vi "fWform to CSV File.vi"(5 "error in (no error)":errorcluster, 6 "Inlude Time Vector":bool, 7 "wForms":waveform(dbl)[](array[waveform]), 9 "CSV Path IN":path) -> (13 "CSV Path OUT":path, 19 "error out":errorcluster)   [LabVIEW 2020, in "TEXT.lvclass"]
uses:
  TEXT.lvclass
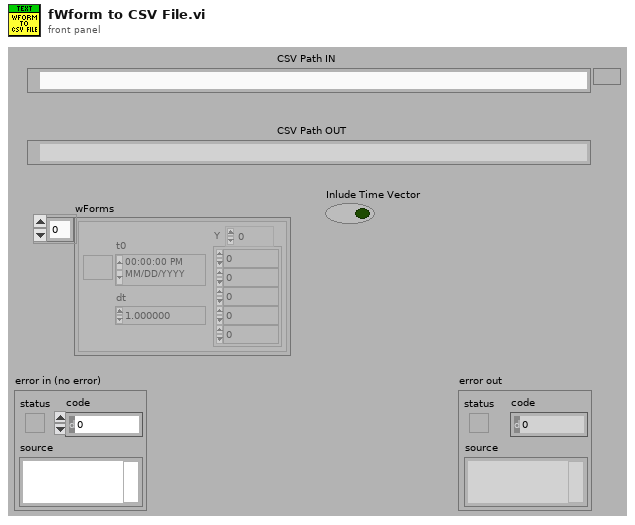
[diagram p1: front panel]
types:
  T1 = enum16{"open", "replace", "create", "open or create", "replace or create", "replace or create with confirmation"}
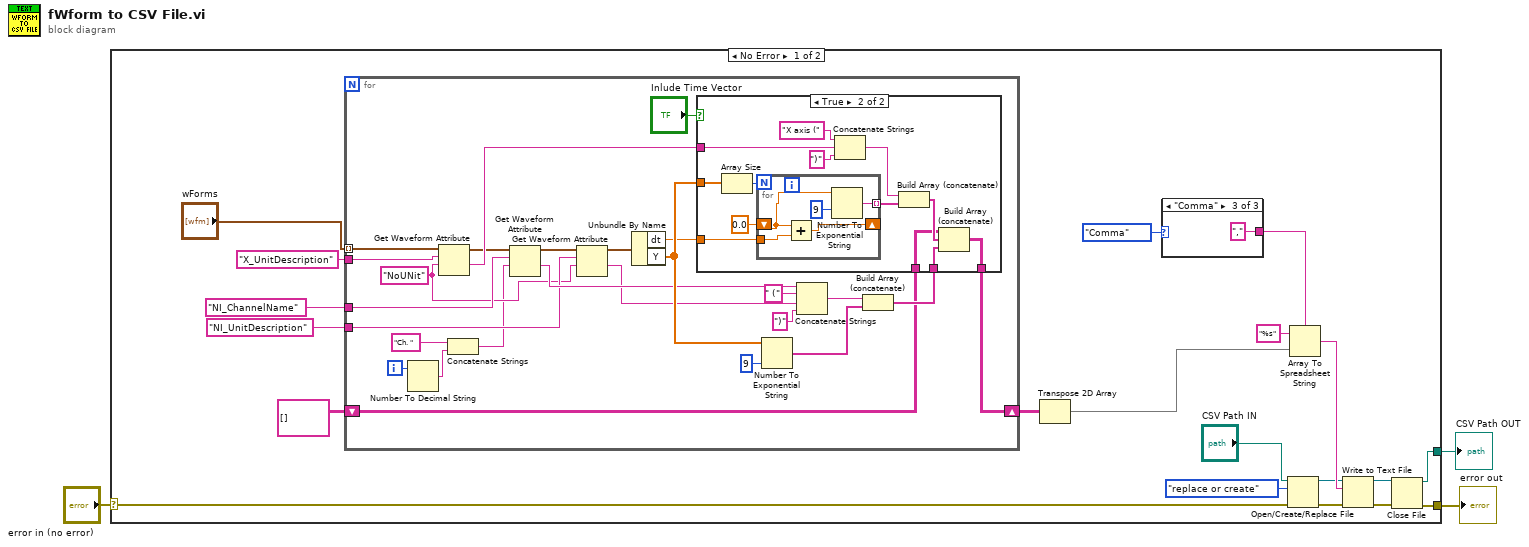
[diagram p0: block diagram]
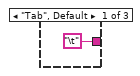
[diagram p2: hidden frame]
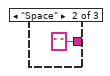
[diagram p3: hidden frame]
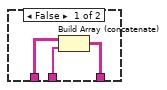
[diagram p4: hidden frame]
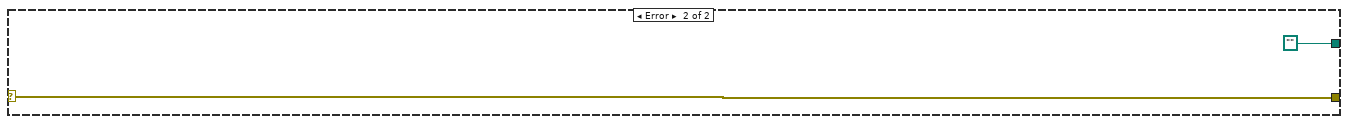
[diagram p5: hidden frame]
diagram:
  n1 = case shown="No Error" "error in (no error)" {
    selector: "error in (no error)" -> [w7 w75]
    tunnel: [w6 w75] -> w2
    tunnel: [w5 path ""] -> w1
    frame No Error {
      n2 = for {
        tunnel: "wForms" -> [w51] mode=indexing
        tunnel: "NI_ChannelName" ("Att - wform Name") -> [w40]
        shift-right: [w46] -> w11
        shift-left: string[][] [] -> [w47]
        tunnel: "X_UnitDescription" ("Att - X unit") -> [w45]
        tunnel: "NI_UnitDescription" ("Att - wform unit") -> [w36]
        i -> [w32]
        w33 = "NoUNit" ("string")
        n3 = Number To Decimal String(number=w32) -> (decimal integer string=w31:string)  [unwired: 1 in]
        n4 = Get Waveform Attribute(5:w33, 6:w45, 7:w51) -> (1:w44:string, 3:w41:waveform(dbl))  [unwired: 1 in, 2 out]
        n5 = Concatenate Strings("Ch. " ("string"), w31) -> (w29:string)
        n6 = Get Waveform Attribute(5:w29, 6:w40, 7:w41) -> (1:w39:string, 3:w38:waveform(dbl))  [unwired: 1 in, 2 out]
        n7 = Get Waveform Attribute(5:w33, 6:w36, 7:w38) -> (1:w35:string, 3:w37:waveform(dbl))  [unwired: 1 in, 2 out]
        n8 = Unbundle By Name(w37) -> ("dt"=w49:dbl, "Y"=w50:dbl[])
        n9 = Number To Exponential String(number=w50, precision (6)=i16 9) -> (E-format string=w52:string[])  [unwired: 2 in]
        n10 = Concatenate Strings(w39, " (" ("string"), w35, ")" ("string")) -> (w34:string)
        n11 = Build Array (concatenate)(w34, w52) -> (w48:string[])
        n12 = case shown="True" "Inlude Time Vector" {
          tunnel: w50 -> [_ w68]
          tunnel: w49 -> [_ w66]
          tunnel: w48 -> [w55 w64]
          tunnel: w47 -> [w54 w62]
          tunnel: [w53 w61] -> w46
          tunnel: w44 -> [_ w57]
          frame False {
            n13 = Build Array (concatenate)(w54, w55) -> (w53:string[][])
          }
          frame True {
            n14 = Array Size(array=w68) -> (size(s)=w67:i32)
            n15 = for {
              N: w67 -> [_]
              shift-right: [w72] -> _
              shift-left: 0.0 -> [w71]
              tunnel: w66 -> [w73]
              tunnel: [w70] -> w56 mode=indexing
              n16 = Add(x=w71, y=w73) -> (x+y=w72:dbl)
              n17 = Number To Exponential String(number=w71, precision (6)=i16 9) -> (E-format string=w70:string)  [unwired: 2 in]
            }
            n18 = Concatenate Strings("X axis (" ("format string"), w57, ")" ("string")) -> (w58:string)
            n19 = Build Array (concatenate)(w58, w56) -> (w63:string[])
            n20 = Build Array (concatenate)(w62, w63, w64) -> (w61:string[][])
          }
        }
      }
      n21 = Transpose 2D Array(2D array=w11) -> (transposed array=w12:string[][])
      n22 = case shown="\"Comma\"" enum16{"Tab", "Space", "Comma"}."Comma" ("Delimiter") {
        tunnel: ["\t" " " ("delimiter (Tab)") "," ("delimiter (Tab)")] -> w20
        frame "Tab", Default {
        }
        frame "Space" {
        }
        frame "Comma" {
        }
      }
      n23 = Open/Create/Replace File(file path (use dialog)="CSV Path IN", error in=w7, operation (0:open)=T1."replace or create") -> (refnum out=w15:refnum<file>, error out=w14:errorcluster)  [unwired: 4 out]
      n24 = Array To Spreadsheet String(delimiter (Tab)=w20, array=w12, 3:"%s" ("format string")) -> (spreadsheet string=w16:string)
      n25 = Write to Text File(file (use dialog)=w15, text=w16, error in=w14) -> (refnum out=w18:refnum<file>, error out=w17:errorcluster)  [unwired: 2 out]
      n26 = Close File(refnum=w18, error in=w17) -> (path=w5:path, error out=w6:errorcluster)
    }
    frame Error {
    }
  }
  "error out" <- w2
  "CSV Path OUT" <- w1
